vi "Convert_static_ARM_line.vi"(10 "sequence line":string[](array[string])) -> (3 "コマンド配列":string[](array[string]))   [LabVIEW 2017]
panel:
  in  "ダミー":string[](array[string])
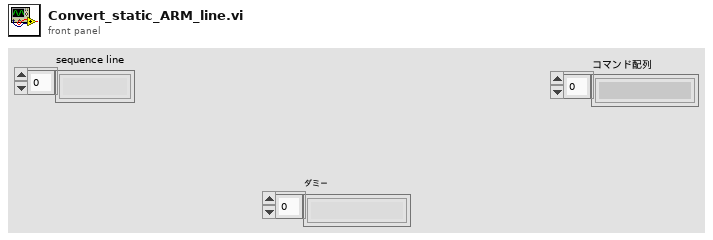
[diagram p1: front panel]
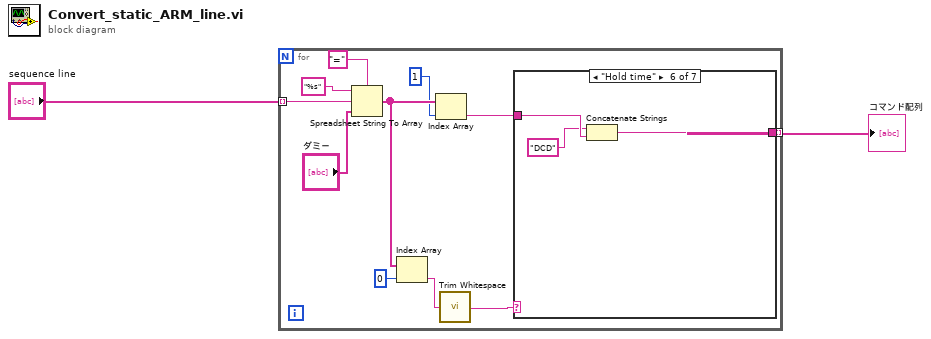
[diagram p0: block diagram]
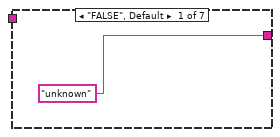
[diagram p2: hidden frame]
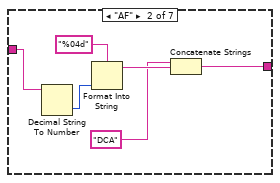
[diagram p3: hidden frame]
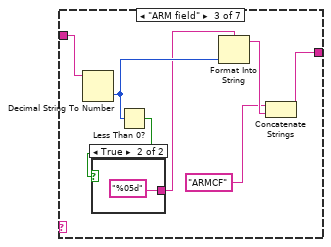
[diagram p4: hidden frame]
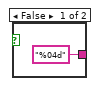
[diagram p5: hidden frame]
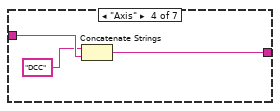
[diagram p6: hidden frame]
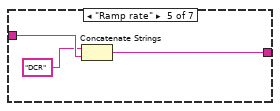
[diagram p7: hidden frame]
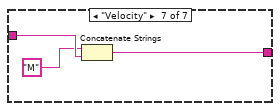
[diagram p8: hidden frame]
diagram:
  n1 = for {
    tunnel: "sequence line" -> [w11] mode=indexing
    tunnel: [w5] -> w1 mode=indexing
    n2 = Spreadsheet String To Array(delimiter (Tab)="=", format string="%s", spreadsheet string=w11, array type (2D Dbl)="ダミー") -> (array=w8:string[])
    n3 = Index Array(array=w8, index=0) -> (element=w4:string)
    n4 = Index Array(array=w8, index=1) -> (element=w6:string)
    n5 = call <vilib>:"Trim Whitespace.vi"("string"=w4) -> ("trimmed string"=w3:string)  [unwired: 1 in]
    n6 = case shown="\"Hold time\"" w3 {
      tunnel: w6 -> [_ w16 w26 w32 w35 w38 w41]
      tunnel: ["unknown" w20 w27 w31 w34 w37 w40] -> w5
      frame "FALSE", Default {
      }
      frame "AF" {
        n7 = Decimal String To Number(string=w16) -> (number=w15:i32)  [unwired: 2 in, 1 out]
        n8 = Format Into String(format string="%04d", w15) -> (resulting string=w18:string)  [unwired: 2 in, 1 out]
        n9 = Concatenate Strings("DCA", w18) -> (w20:string)
      }
      frame "ARM field" {
        n10 = Decimal String To Number(string=w26) -> (number=w24:i32)  [unwired: 2 in, 1 out]
        n11 = Less Than 0?(x=w24) -> (x < 0?=w22:bool)
        n12 = case shown="TRUE" w22 {
          tunnel: ["%04d" "%05d"] -> w21
          frame False {
          }
          frame True {
          }
        }
        n13 = Format Into String(format string=w21, w24) -> (resulting string=w25:string)  [unwired: 2 in, 1 out]
        n14 = Concatenate Strings("ARMCF", w25) -> (w27:string)
      }
      frame "Axis" {
        n15 = Concatenate Strings("DCC", w32) -> (w31:string)
      }
      frame "Ramp rate" {
        n16 = Concatenate Strings("DCR", w35) -> (w34:string)
      }
      frame "Hold time" {
        n17 = Concatenate Strings("DCD", w38) -> (w37:string)
      }
      frame "Velocity" {
        n18 = Concatenate Strings("M", w41) -> (w40:string)
      }
    }
  }
  "コマンド配列" <- w1
